vi "Destroy.vi"(8 "error in (no error)":errorcluster, 11 "Excel refnum":T1) -> (0 "error out":errorcluster, 3 "file path":path)   [LabVIEW 2020, in "NI_ExcelFile.lvlib"]
doc: "Closes the reference to the .xlsx file that you created or opened with the Create VI. Error I/O operates uniquely in this VI, which closes the .xlsx file regardless of whether an error occurred in a preceding operation. This ensures that the .xlsx file is closed and temporary files are deleted correctly.\n \nExcel refnum: Specifies a reference to the .xlsx file on which to perform the operation. Use the Create VI to create or open the refnum.\n\nerror in: describes error conditions that occur before this node runs. This input provides standard error in functionality.\n\nfile path: Returns the absolute path of the .xlsx file.\n\nerror out: contains error information. This output provides standard error out functionality."
uses:
  <vilib>/express/express shared/NI_ExcelFile/NI_ExcelFile.lvlib
  <vilib>/express/express shared/NI_ExcelFile/Ctrls/ExcelRefnum.ctl
  <vilib>/express/express shared/NI_ExcelFile/Ctrls/MainData.ctl
  <vilib>/express/express shared/NI_ExcelFile/Ctrls/StreamMode.ctl
  <vilib>/express/express shared/NI_ExcelFile/Ctrls/TimeColumnMode.ctl
  <vilib>/express/express shared/NI_ExcelFile/Ctrls/FileAttribute.ctl
  <vilib>/express/express shared/NI_ExcelFile/Ctrls/Columns.ctl
  <vilib>/express/express shared/NI_ExcelFile/Ctrls/ColumnInfo.ctl
  <vilib>/express/express shared/NI_ExcelFile/Ctrls/DataType.ctl
  <vilib>/express/express shared/NI_ExcelFile/Ctrls/wd_recordInfo.ctl
  <vilib>/express/express shared/NI_ExcelFile/Ctrls/disk_TemplateFile.ctl
  <vilib>/express/express shared/NI_ExcelFile/Ctrls/meta_file.ctl
  <vilib>/express/express shared/NI_ExcelFile/Ctrls/meta_Block.ctl
  <vilib>/express/express shared/NI_ExcelFile/Ctrls/meta_BlockType.ctl
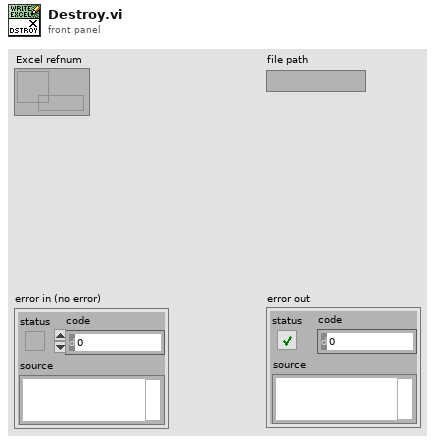
[diagram p1: front panel]
types:
  T1 = typedef "NI_ExcelFile.lvlib/ExcelRefnum.ctl" = refnum<data-value>
  T2 = typedef "NI_ExcelFile.lvlib/MainData.ctl" = cluster{"TargetFile":path, "StreamMode":T3, "Append?":bool, "ChunkSize":u64, "TimeColumnMode":T4, "TimestampFormat":string, "AbsoluteTime?":bool, "FileAttribute ":T5, "Column":T6, "FileRef":refnum<k1>, "MemoryRef":refnum<data-value>[], "RecordInfo":T9[], " ChannelPreviousInfo":u32[], "ChannelFirstRecord":u32[], "PredefinedFormattedValueLength":i64, "DiskTemplate":T10}
  T3 = typedef "NI_ExcelFile.lvlib/StreamMode.ctl" = enum16{"File", "Memory"}
  T4 = typedef "NI_ExcelFile.lvlib/TimeColumnMode.ctl" = enum16{"Empty", "OnePerCh", "One"}
  T5 = typedef "NI_ExcelFile.lvlib/FileAttribute.ctl" = cluster{"Creator":string, "Title":string, "SheetName":string}
  T6 = typedef "NI_ExcelFile.lvlib/Columns.ctl" = T7[]
  T7 = typedef "NI_ExcelFile.lvlib/ColumnInfo.ctl" = cluster{"Header":string, "Format":string, "DataType":T8, "Length":u64}
  T8 = typedef "NI_ExcelFile.lvlib/DataType.ctl" = enum16{"DDT", "WFM", "Array of STR", "Array of DBL", "Array of I8", "Array of I16", "Array of I32", "Array of I64", "Array of SGL", "Array of U8", "Array of U16", "Array of U32", "Array of U64", "Array of Time"}
  T9 = typedef "NI_ExcelFile.lvlib/wd_recordInfo.ctl" = cluster{"ChannelIndex":u32, "StartIndex":u64, "Length":u64, "Previous":i32, "Next":i32}
  T10 = typedef "NI_ExcelFile.lvlib/disk_TemplateFile.ctl" = cluster{"XMLRef":refnum<file>[], "ZipPath":path, "MetaFile":T11, "TempFolder":path}
  T11 = typedef "NI_ExcelFile.lvlib/meta_file.ctl" = cluster{"Ref":refnum<file>, "NextRow":i32, "NextPosition":i64, "Block":T12[]}
  T12 = typedef "NI_ExcelFile.lvlib/meta_Block.ctl" = cluster{"Version":u16, "Type":T13, "Length":i32, "Data":string}
  T13 = typedef "NI_ExcelFile.lvlib/meta_BlockType.ctl" = enum16{"NITag", "File", "Column"}
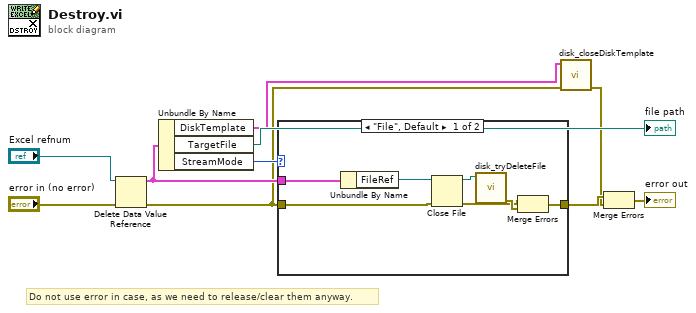
[diagram p0: block diagram]
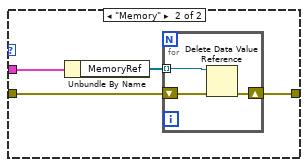
[diagram p2: hidden frame]
diagram:
  # "Do not use error in case, as we need to release/clear them anyway."
  n1 = Delete Data Value Reference(data value reference="Excel refnum", error in="error in (no error)") -> (data value=w7:T2, error out=w3:errorcluster)
  n2 = Unbundle By Name(w7) -> ("DiskTemplate"=w6:T10, "TargetFile"=→"file path":path, "StreamMode"=w8:T3)
  n3 = case shown="\"File\", Default" w8 {
    tunnel: w7 -> [w17 w21]
    tunnel: [w13 w19] -> w2
    tunnel: w3 -> [w14 w18]
    frame "File", Default {
      n4 = Unbundle By Name(w17) -> ("FileRef"=w16:refnum<k1>)
      n5 = Close File(refnum=w16, error in=w14) -> (path=w15:path, error out=w11:errorcluster)
      n6 = call <vilib>:"disk_tryDeleteFile.vi"("path"=w15) -> ("error out"=w12:errorcluster)  [unwired: 10 in]
      n7 = Merge Errors(w11, w12) -> (w13:errorcluster)
    }
    frame "Memory" {
      n8 = Unbundle By Name(w21) -> ("MemoryRef"=w20:refnum<data-value>[])
      n9 = for {
        tunnel: w20 -> [w24] mode=indexing
        shift-right: [w22] -> w19
        shift-left: w18 -> [w23]
        n10 = Delete Data Value Reference(data value reference=w24, error in=w23) -> (error out=w22:errorcluster)  [unwired: 1 out]
      }
    }
  }
  n11 = call <vilib>:"disk_closeDiskTemplate.vi"("error in (no error)"=w3, "DiskTemplate in"=w6) -> ("error out"=w1:errorcluster)  [unwired: 9 in]
  n12 = Merge Errors(w2, w1) -> (→"error out":errorcluster)
